vi "sub vi - send mail with attach v5.vi"(0 "TO:":string, 1 "subject":string, 5 "from":string, 7 "out going server":string, 9 "message":string, 11 "username":string, 12 "password":string, 13 "Attachements":path[](array[path])) -> (15 "error out":errorcluster)   [LabVIEW 2013]
uses:
  <vilib>/Utility/SMTP/NI_SMTPEmail.lvlib
panel:
  in  "Tab Control":enum32{"Page 1", "Page 2"}(tab)
  in  "Mail To:":string[](array[string])
  # "SENDING MAIL"
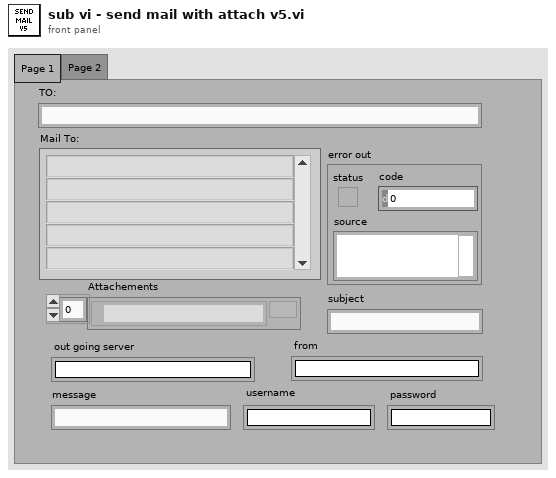
[diagram p1: front panel]
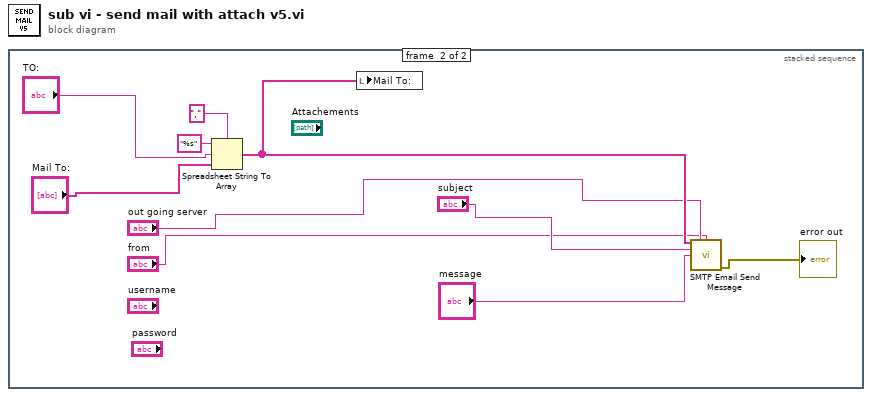
[diagram p0: block diagram]
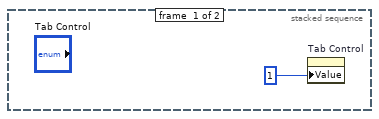
[diagram p2: hidden frame]
diagram:
  n1 = stacked-sequence {
    frame #0 {
      n2 = property on="Tab Control" class="TabCtl (strict)"("Value"=1) -> ()  [unwired: 2 in, 2 out]
    }
    frame #1 {
      n3 = Spreadsheet String To Array(delimiter (Tab)=",", format string="%s", spreadsheet string="TO:", array type (2D Dbl)="Mail To:") -> (array=w6:string[])
      n4 = local write "Mail To:"(w6) -> ()
      n5 = call <vilib>:"SMTP Email Send Message.vi"("recipients"=w6, "mail server"="out going server", "return address"="from", "subject ([No Subject])"="subject", "message"="message") -> ("error out"=→"error out":errorcluster)  [unwired: 9 in, 1 out]
    }
  }
